vi "Value Read.vi"(7 "Read Values":T1=100 items=["Device Type"=100, "Hardware Version"=101, "Serial Number"=102, "Firmware Version"=103, "Device Status"=104, "Error Number"=105, "Error Instance"=106, "Error Parameter"=107, "Save Data to Flash"=108, "Flash Status"=109, "Object Temperature"=1000, "Sink Temperature"=1001, "Target Obj Temperature"=1010, "Nominal Obj Temperature"=1011, "Thermal Power Mod Current"=1012, "Actual Output Current"=1020, "Actual Output Voltage"=1021, "Relative Cooling Power"=1100, "Nominal Fan Speed"=1101, "Actual Fan Speed"=1102, "Fan PWM Level"=1103, "PID Lower Limitation"=1030, "PID Upper Limitation"=1031, "PID Control Variable"=1032, "Obj Sensor Raw ADC Val"=1040, "Sink Sensor Raw ADC Val"=1041, "Object Sensor Resistance"=1042, "Sink Sensor Resistance"=1043, "Driver Input Voltage"=1060, "10V Internal Supply"=1061, "3.3V Internal Supply"=1062, "Base Plate Temperature"=1063, "Error Number"=1070, "Error Instance"=1071, "Error Parameter"=1072, "Temperature is Stable"=1200], 9 "Sequence":string="0000", 10 "Instance":string="01", 11 "Address":u8) -> (2 "hex integer string":string)   [LabVIEW 2014, in "Meerstetter Lib.lvlib" / "Meerstetter TEC.lvclass"]
doc: "Provides a string for sending to a serial port given a particular address, sequence and instance number as well as the command."
uses:
  Meerstetter TEC.lvclass
  Controls/Read Parameters.ctl
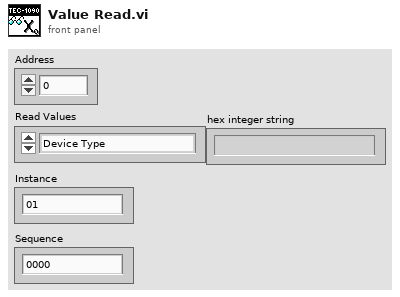
[diagram p1: front panel]
types:
  T1 = typedef "Meerstetter Lib.lvlib/Meerstetter TEC.lvclass/Read Parameters.ctl" = u16
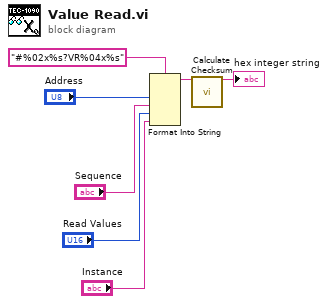
[diagram p0: block diagram]
diagram:
  n1 = Format Into String(format string="#%02x%s?VR%04x%s", "Address", "Sequence", "Read Values", "Instance") -> (resulting string=w5:string)  [unwired: 2 in, 1 out]
  n2 = call "Calculate Checksum.vi"("Message"=w5) -> ("MSG"=→"hex integer string":string)  [unwired: 11 in, 3 out]
